vi "日志、报警信息存储 (子VI).vi"() -> ()   [LabVIEW 2016, in "德润超标留样.lvlib"]
panel:
  out "采样器状态":T1
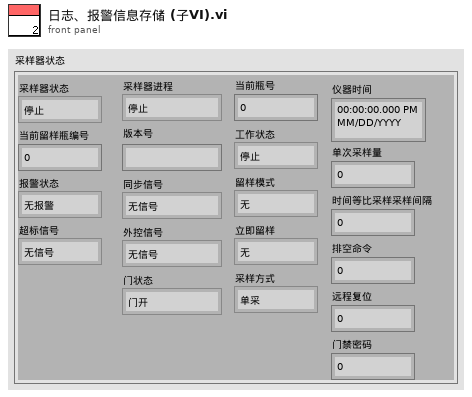
[diagram p1: front panel]
types:
  T1 = cluster{"采样器状态":enum16{"停止", "运行"}, "当前留样瓶编号":u16, "报警状态":enum16{"无报警", "缺水报警"}, "超标信号":enum16{"无信号", "超标信号"}, "采样器进程":enum16{"停止", "待机", "定位校正", "移除瓶盖", "采样瓶排空", "管路润洗", "管存", "进样", "瓶盖密封", "管路排空", "调整采样位置", "采样结束", "采样瓶润洗", "瓶润洗排空"}, "版本号":string, "同步信号":enum16{"无信号", "同步信号"}, "外控信号":enum16{"无信号", "外控信号"}, "门状态":enum16{"门开", "门关"}, "当前瓶号":u16, "工作状态":enum16{"停止", "采样中"}, "留样模式":enum16{"无", "定时留样", "时间等比例", "超标留样", "同步留样", "外控留样"}, "立即留样":enum16{"无", "远程留样"}, "采样方式":enum16{"单采", "双重"}, "仪器时间":timestamp, "单次采样量":u16, "时间等比采样采样间隔":u16, "排空命令":u16, "远程复位":u16, "门禁密码":u16}
  T2 = cluster{"时间标识":timestamp, "设备":string, "日志信息":string, "流程参数":string}
  T3 = cluster{"时间标识":timestamp, "设备":string, "日志信息":string}
  T4 = enum16{"停止", "待机", "定位校正", "移除瓶盖", "采样瓶排空", "管路润洗", "管存", "进样", "瓶盖密封", "管路排空", "调整采样位置", "采样结束", "采样瓶润洗", "瓶润洗排空"}
  T5 = enum16{"无", "定时留样", "时间等比例", "超标留样", "同步留样", "外控留样"}
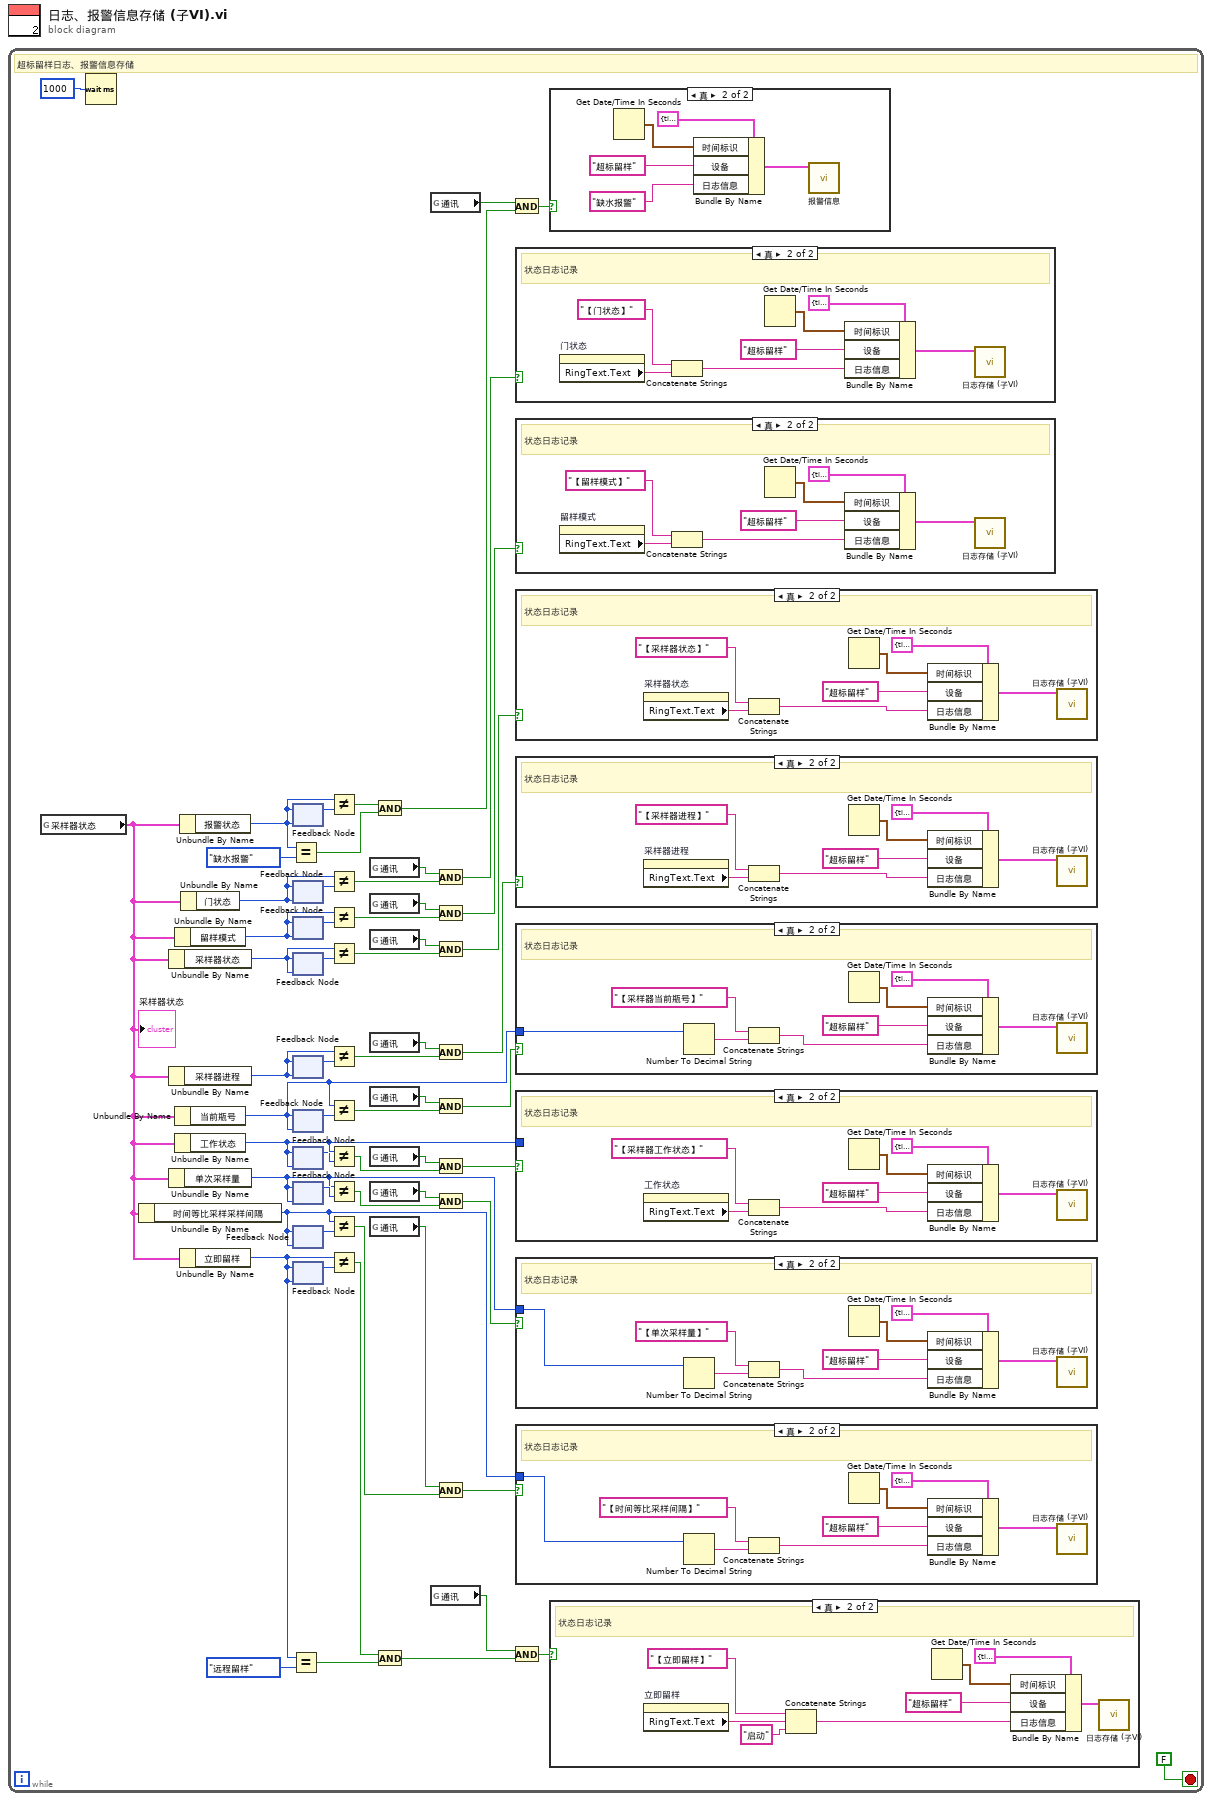
[diagram p0: block diagram]
diagram:
  n1 = while {
    stop <- FALSE stop-if-true
    # "超标留样日志、报警信息存储"
    n2 = global read "超标留样全局.vi" "采样器状态"() -> (w2:T1)
    "采样器状态" <- w2
    n3 = Wait (ms)(milliseconds to wait=u32 1000 ("等待时间（毫秒）")) -> ()  [unwired: 1 out]
    n4 = Unbundle By Name(w2) -> ("时间等比采样采样间隔"=w10:u16)
    n5 = Unbundle By Name(w2) -> ("采样器状态"=w55:enum16{"停止", "运行"})
    n6 = Unbundle By Name(w2) -> ("采样器进程"=w50:T4)
    n7 = Unbundle By Name(w2) -> ("单次采样量"=w33:u16)
    n8 = Unbundle By Name(w2) -> ("留样模式"=w17:T5)
    n9 = Unbundle By Name(w2) -> ("当前瓶号"=w43:u16)
    n10 = Unbundle By Name(w2) -> ("工作状态"=w42:enum16{"停止", "采样中"})
    n11 = Unbundle By Name(w2) -> ("报警状态"=w26:enum16{"无报警", "缺水报警"})
    n12 = Unbundle By Name(w2) -> ("立即留样"=w8:enum16{"无", "远程留样"})
    n13 = Unbundle By Name(w2) -> ("门状态"=w22:enum16{"门开", "门关"})
    n14 = Equal?(x=w26, y=enum16{"无报警", "缺水报警"}."缺水报警" ("报警状态")) -> (x = y?=w25:bool)
    n15 = Equal?(x=w8, y=enum16{"无", "远程留样"}."远程留样" ("立即留样")) -> (x = y?=w9:bool)
    n16 = feedback #1(w26) -> (w31:enum16{"无报警", "缺水报警"})
    n17 = feedback-in #1(w26) -> ()
    n18 = feedback #2(w22) -> (w23:enum16{"门开", "门关"})
    n19 = feedback-in #2(w22) -> ()
    n20 = feedback #3(w17) -> (w16:T5)
    n21 = feedback-in #3(w17) -> ()
    n22 = feedback #4(w55) -> (w56:enum16{"停止", "运行"})
    n23 = feedback-in #4(w55) -> ()
    n24 = feedback #5(w50) -> (w49:T4)
    n25 = feedback-in #5(w50) -> ()
    n26 = feedback #6(w43) -> (w46:u16)
    n27 = feedback-in #6(w43) -> ()
    n28 = feedback #7(w42) -> (w39:enum16{"停止", "采样中"})
    n29 = feedback-in #7(w42) -> ()
    n30 = feedback #8(w33) -> (w36:u16)
    n31 = feedback-in #8(w33) -> ()
    n32 = feedback #9(w10) -> (w12:u16)
    n33 = feedback-in #9(w10) -> ()
    n34 = feedback #10(w8) -> (w5:enum16{"无", "远程留样"})
    n35 = feedback-in #10(w8) -> ()
    n36 = Not Equal?(x=w26, y=w31) -> (x != y?=w29:bool)
    n37 = Not Equal?(x=w22, y=w23) -> (x != y?=w24:bool)
    n38 = Not Equal?(x=w17, y=w16) -> (x != y?=w15:bool)
    n39 = Not Equal?(x=w55, y=w56) -> (x != y?=w57:bool)
    n40 = Not Equal?(x=w50, y=w49) -> (x != y?=w48:bool)
    n41 = Not Equal?(x=w43, y=w46) -> (x != y?=w47:bool)
    n42 = Not Equal?(x=w42, y=w39) -> (x != y?=w38:bool)
    n43 = Not Equal?(x=w33, y=w36) -> (x != y?=w37:bool)
    n44 = Not Equal?(x=w10, y=w12) -> (x != y?=w11:bool)
    n45 = Not Equal?(x=w8, y=w5) -> (x != y?=w6:bool)
    n46 = global read "超标留样全局.vi" "通讯"() -> (w21:bool)
    n47 = global read "超标留样全局.vi" "通讯"() -> (w18:bool)
    n48 = global read "超标留样全局.vi" "通讯"() -> (w54:bool)
    n49 = global read "超标留样全局.vi" "通讯"() -> (w51:bool)
    n50 = global read "超标留样全局.vi" "通讯"() -> (w45:bool)
    n51 = global read "超标留样全局.vi" "通讯"() -> (w40:bool)
    n52 = global read "超标留样全局.vi" "通讯"() -> (w35:bool)
    n53 = global read "超标留样全局.vi" "通讯"() -> (w13:bool)
    n54 = And(x=w29, y=w25) -> (x .and. y?=w28:bool)
    n55 = And(x=w6, y=w9) -> (x .and. y?=w7:bool)
    n56 = global read "超标留样全局.vi" "通讯"() -> (w32:bool)
    n57 = global read "超标留样全局.vi" "通讯"() -> (w4:bool)
    n58 = And(x=w21, y=w24) -> (x .and. y?=w20:bool)
    n59 = And(x=w18, y=w15) -> (x .and. y?=w19:bool)
    n60 = And(x=w54, y=w57) -> (x .and. y?=w53:bool)
    n61 = And(x=w51, y=w48) -> (x .and. y?=w52:bool)
    n62 = And(x=w45, y=w47) -> (x .and. y?=w44:bool)
    n63 = And(x=w40, y=w38) -> (x .and. y?=w41:bool)
    n64 = And(x=w35, y=w37) -> (x .and. y?=w34:bool)
    n65 = And(x=w13, y=w11) -> (x .and. y?=w14:bool)
    n66 = And(x=w32, y=w28) -> (x .and. y?=w30:bool)
    n67 = And(x=w4, y=w7) -> (x .and. y?=w3:bool)
    n68 = case shown="真" w20 {
      frame False {
      }
      frame True {
        # "状态日志记录"
        n69 = property on="门状态" class="Enum (严格)"() -> ("RingText.Text"=w83:string)  [unwired: 2 in, 2 out]
        n70 = Concatenate Strings("【门状态】" ("日志信息"), w83) -> (w89:string)
        n71 = Get Date/Time In Seconds() -> (seconds since 1Jan1904=w86:timestamp)
        n72 = Bundle By Name(cluster=T2 {"时间标识"=timestamp(0 s since 1904-01-01), "设备"="", "日志信息"="", "流程参数"=""} ("data in"), "时间标识"=w86, "设备"="超标留样", "日志信息"=w89) -> (w85:T2)
        n73 = call "日志存储 (子VI).vi"("data in"=w85) -> ()  [unwired: 11 in]
      }
    }
    n74 = case shown="真" w19 {
      frame False {
      }
      frame True {
        # "状态日志记录"
        n75 = property on="留样模式" class="Enum (严格)"() -> ("RingText.Text"=w76:string)  [unwired: 2 in, 2 out]
        n76 = Concatenate Strings("【留样模式】" ("日志信息"), w76) -> (w82:string)
        n77 = Get Date/Time In Seconds() -> (seconds since 1Jan1904=w79:timestamp)
        n78 = Bundle By Name(cluster=T2 {"时间标识"=timestamp(0 s since 1904-01-01), "设备"="", "日志信息"="", "流程参数"=""} ("data in"), "时间标识"=w79, "设备"="超标留样", "日志信息"=w82) -> (w78:T2)
        n79 = call "日志存储 (子VI).vi"("data in"=w78) -> ()  [unwired: 11 in]
      }
    }
    n80 = case shown="真" w53 {
      frame False {
      }
      frame True {
        # "状态日志记录"
        n81 = property on="采样器状态" class="Enum (严格)"() -> ("RingText.Text"=w125:string)  [unwired: 2 in, 2 out]
        n82 = Concatenate Strings("【采样器状态】" ("日志信息"), w125) -> (w131:string)
        n83 = Get Date/Time In Seconds() -> (seconds since 1Jan1904=w128:timestamp)
        n84 = Bundle By Name(cluster=T2 {"时间标识"=timestamp(0 s since 1904-01-01), "设备"="", "日志信息"="", "流程参数"=""} ("data in"), "时间标识"=w128, "设备"="超标留样", "日志信息"=w131) -> (w127:T2)
        n85 = call "日志存储 (子VI).vi"("data in"=w127) -> ()  [unwired: 11 in]
      }
    }
    n86 = case shown="真" w52 {
      frame False {
      }
      frame True {
        # "状态日志记录"
        n87 = property on="采样器进程" class="Enum (严格)"() -> ("RingText.Text"=w118:string)  [unwired: 2 in, 2 out]
        n88 = Concatenate Strings("【采样器进程】" ("日志信息"), w118) -> (w124:string)
        n89 = Get Date/Time In Seconds() -> (seconds since 1Jan1904=w121:timestamp)
        n90 = Bundle By Name(cluster=T2 {"时间标识"=timestamp(0 s since 1904-01-01), "设备"="", "日志信息"="", "流程参数"=""} ("data in"), "时间标识"=w121, "设备"="超标留样", "日志信息"=w124) -> (w120:T2)
        n91 = call "日志存储 (子VI).vi"("data in"=w120) -> ()  [unwired: 11 in]
      }
    }
    n92 = case shown="真" w44 {
      tunnel: w43 -> [_ w111]
      frame False {
      }
      frame True {
        # "状态日志记录"
        n93 = Number To Decimal String(number=w111) -> (decimal integer string=w110:string)  [unwired: 1 in]
        n94 = Concatenate Strings("【采样器当前瓶号】" ("日志信息"), w110) -> (w117:string)
        n95 = Get Date/Time In Seconds() -> (seconds since 1Jan1904=w114:timestamp)
        n96 = Bundle By Name(cluster=T2 {"时间标识"=timestamp(0 s since 1904-01-01), "设备"="", "日志信息"="", "流程参数"=""} ("data in"), "时间标识"=w114, "设备"="超标留样", "日志信息"=w117) -> (w113:T2)
        n97 = call "日志存储 (子VI).vi"("data in"=w113) -> ()  [unwired: 11 in]
      }
    }
    n98 = case shown="真" w41 {
      tunnel: w42 -> [_ _]
      frame False {
      }
      frame True {
        # "状态日志记录"
        n99 = property on="工作状态" class="Enum (严格)"() -> ("RingText.Text"=w103:string)  [unwired: 2 in, 2 out]
        n100 = Concatenate Strings("【采样器工作状态】" ("日志信息"), w103) -> (w109:string)
        n101 = Get Date/Time In Seconds() -> (seconds since 1Jan1904=w106:timestamp)
        n102 = Bundle By Name(cluster=T2 {"时间标识"=timestamp(0 s since 1904-01-01), "设备"="", "日志信息"="", "流程参数"=""} ("data in"), "时间标识"=w106, "设备"="超标留样", "日志信息"=w109) -> (w105:T2)
        n103 = call "日志存储 (子VI).vi"("data in"=w105) -> ()  [unwired: 11 in]
      }
    }
    n104 = case shown="真" w34 {
      tunnel: w33 -> [_ w96]
      frame False {
      }
      frame True {
        # "状态日志记录"
        n105 = Number To Decimal String(number=w96) -> (decimal integer string=w95:string)  [unwired: 1 in]
        n106 = Concatenate Strings("【单次采样量】" ("日志信息"), w95) -> (w102:string)
        n107 = Get Date/Time In Seconds() -> (seconds since 1Jan1904=w99:timestamp)
        n108 = Bundle By Name(cluster=T2 {"时间标识"=timestamp(0 s since 1904-01-01), "设备"="", "日志信息"="", "流程参数"=""} ("data in"), "时间标识"=w99, "设备"="超标留样", "日志信息"=w102) -> (w98:T2)
        n109 = call "日志存储 (子VI).vi"("data in"=w98) -> ()  [unwired: 11 in]
      }
    }
    n110 = case shown="真" w14 {
      tunnel: w10 -> [_ w69]
      frame False {
      }
      frame True {
        # "状态日志记录"
        n111 = Number To Decimal String(number=w69) -> (decimal integer string=w68:string)  [unwired: 1 in]
        n112 = Concatenate Strings("【时间等比采样间隔】" ("日志信息"), w68) -> (w75:string)
        n113 = Get Date/Time In Seconds() -> (seconds since 1Jan1904=w72:timestamp)
        n114 = Bundle By Name(cluster=T2 {"时间标识"=timestamp(0 s since 1904-01-01), "设备"="", "日志信息"="", "流程参数"=""} ("data in"), "时间标识"=w72, "设备"="超标留样", "日志信息"=w75) -> (w71:T2)
        n115 = call "日志存储 (子VI).vi"("data in"=w71) -> ()  [unwired: 11 in]
      }
    }
    n116 = case shown="真" w30 {
      frame False {
      }
      frame True {
        n117 = Get Date/Time In Seconds() -> (seconds since 1Jan1904=w94:timestamp)
        n118 = Bundle By Name(cluster=T3 {"时间标识"=timestamp(0 s since 1904-01-01), "设备"="", "日志信息"=""} ("data in"), "时间标识"=w94, "设备"="超标留样", "日志信息"="缺水报警") -> (w90:T3)
        n119 = call "报警信息.vi"("data in"=w90) -> ()  [unwired: 10 in, 1 out]
      }
    }
    n120 = case shown="真" w3 {
      frame False {
      }
      frame True {
        # "状态日志记录"
        n121 = property on="立即留样" class="Enum (严格)"() -> ("RingText.Text"=w61:string)  [unwired: 2 in, 2 out]
        n122 = Concatenate Strings("【立即留样】" ("日志信息"), w61, "启动" ("字符串")) -> (w67:string)
        n123 = Get Date/Time In Seconds() -> (seconds since 1Jan1904=w64:timestamp)
        n124 = Bundle By Name(cluster=T2 {"时间标识"=timestamp(0 s since 1904-01-01), "设备"="", "日志信息"="", "流程参数"=""} ("data in"), "时间标识"=w64, "设备"="超标留样", "日志信息"=w67) -> (w63:T2)
        n125 = call "日志存储 (子VI).vi"("data in"=w63) -> ()  [unwired: 11 in]
      }
    }
  }
